vi "Read Value.vi"(8 "error in (no error)":errorcluster, 10 "Trace":i16=1, 11 "VISA Resource Name":refnum<visa-resource-name>) -> (0 "error out":errorcluster, 2 "Value":dbl format="%.4e", 3 "VISA Resource Name Out":refnum<visa-resource-name>)   [LabVIEW 2015]
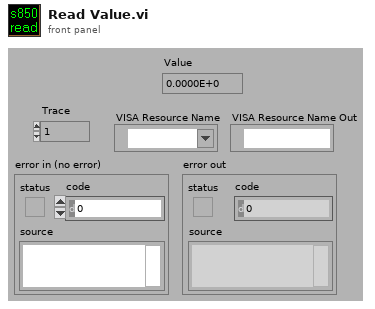
[diagram p1: front panel]
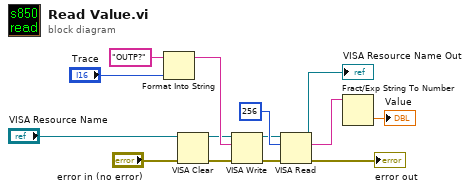
[diagram p0: block diagram]
diagram:
  n1 = Format Into String(initial string="OUTP?", "Trace") -> (resulting string=w8:string)  [unwired: 2 in, 1 out]
  n2 = VISA Clear(VISA resource name="VISA Resource Name", error in (no error)="error in (no error)") -> (VISA resource name out=w5:refnum<visa-resource-name>, error out=w7:errorcluster)
  n3 = VISA Write(VISA resource name=w5, write buffer=w8, error in (no error)=w7) -> (VISA resource name out=w4:refnum<visa-resource-name>, error out=w10:errorcluster)  [unwired: 1 out]
  n4 = VISA Read(VISA resource name=w4, byte count=u32 256, error in (no error)=w10) -> (VISA resource name out=→"VISA Resource Name Out":refnum<visa-resource-name>, read buffer=w3:string, error out=→"error out":errorcluster)  [unwired: 1 out]
  n5 = Fract/Exp String To Number(string=w3) -> (number=→"Value":dbl)  [unwired: 4 out]
